vi "ACT_ServoControl.vi"(2 "y 2":dbl, 3 "y":i32) -> (0 "String":string)   [LabVIEW 2011]
doc: "This vi turns an array of boolean values into the corresponding 8-bit number in a way that a serial port understands. That is, converting a boolean array (1001) to a number (9) then converting that number to a string \"9\". To a serial read, \"9\" is actually a code number (39 in hex) which is not the decimal value 9 (actually it is 57 in base 10). This vi converts the boolean array representing the value 9 into a string (not available in Windows) which when decoded is actually the value 9 (09 in hex, which is 9 in base 10)."
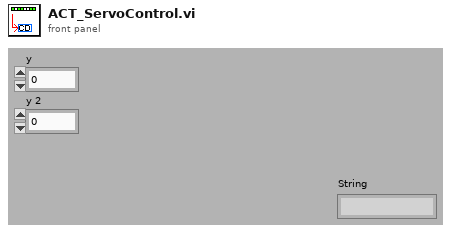
[diagram p1: front panel]
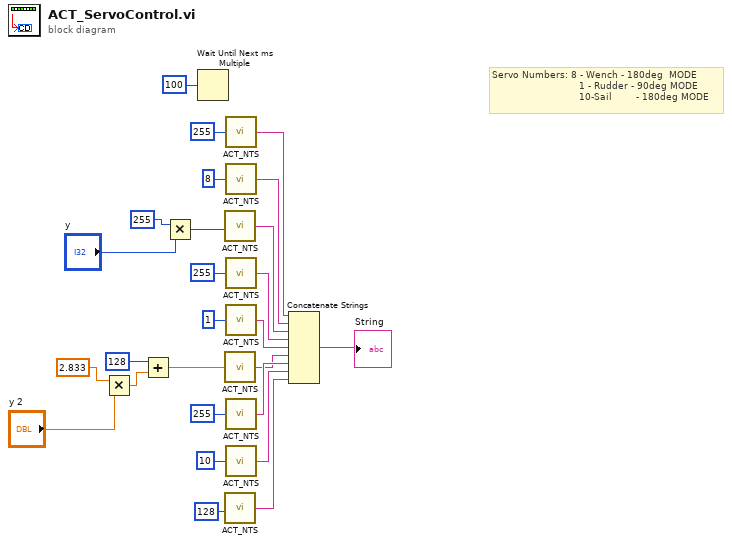
[diagram p0: block diagram]
diagram:
  # "Servo Numbers: 8 - Wench - 180deg  MODE\n                             1 - Rudder - 90deg MODE\n                             10-Sail        - 180deg MODE"
  n1 = Multiply(x=2.833, y="y 2") -> (x*y=w7:dbl)
  n2 = Add(x=128, y=w7) -> (x+y=w6:dbl)
  n3 = Multiply(x=255, y="y") -> (x*y=w4:i32)
  n4 = Wait Until Next ms Multiple(millisecond multiple=u32 100) -> ()  [unwired: 1 out]
  n5 = call "ACT_NTS.vi"("number IN"=w4) -> ("string OUT"=w14:string)
  n6 = call "ACT_NTS.vi"("number IN"=w6) -> ("string OUT"=w11:string)
  n7 = call "ACT_NTS.vi"("number IN"=128) -> ("string OUT"=w19:string)
  n8 = call "ACT_NTS.vi"("number IN"=u8 255) -> ("string OUT"=w16:string)
  n9 = call "ACT_NTS.vi"("number IN"=u8 8) -> ("string OUT"=w15:string)
  n10 = call "ACT_NTS.vi"("number IN"=u8 255) -> ("string OUT"=w13:string)
  n11 = call "ACT_NTS.vi"("number IN"=u8 1) -> ("string OUT"=w12:string)
  n12 = call "ACT_NTS.vi"("number IN"=u8 255) -> ("string OUT"=w21:string)
  n13 = call "ACT_NTS.vi"("number IN"=u8 10) -> ("string OUT"=w20:string)
  n14 = Concatenate Strings(w16, w15, w14, w13, w12, w11, w21, w20, w19) -> (→"String":string)
